vi "Convert Unit (1D-Array).vi"(0 "Data in":dbl[](array[numeric]), 1 "unit":u16) -> (6 "Data out":dbl[](array[numeric]))   [LabVIEW 2019]
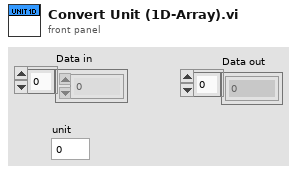
[diagram p1: front panel]
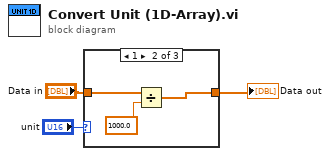
[diagram p0: block diagram]
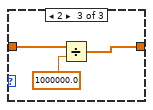
[diagram p3: hidden frame]
diagram:
  n1 = case shown="1" "unit" {
    tunnel: [w4 w7 w10] -> w1
    tunnel: "Data in" -> [w4 w6 w9]
    frame 0, Default {
    }
    frame 1 {
      n2 = Divide(x=w6, y=1000.0) -> (x/y=w7:dbl[])
    }
    frame 2 {
      n3 = Divide(x=w9, y=1000000.0) -> (x/y=w10:dbl[])
    }
  }
  "Data out" <- w1
